vi "Obtain Session.vi"(0 "Listener ID ()":string, 2 "REx Command":refnum<class "REx Command - Root.lvclass">, 11 "error in (no error)":errorcluster) -> (4 "Listener Session Handle":T1, 6 "REx Command Received":refnum<user-event>, 8 "created new?":bool, 15 "error out":errorcluster)   [LabVIEW 2012, in "REx.lvlib" / "Local Listener Session.lvclass"]
doc: "This function initializes the measurement\n\nPass the function a name to obtain an active measurement handle"
uses:
  Local Listener Session.lvclass
  Typedefs/Session Handle.ctl
  REx Command Root/REx Command - Root.lvclass
  Local Listener Session.lvclass/Local Listener Session.ctl
  Utilities/initialize Session Data.vi
  <userlib>/_Session Fwk/Session - Root.lvclass
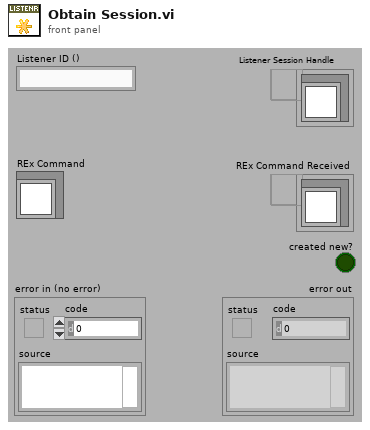
[diagram p1: front panel]
types:
  T1 = typedef "REx.lvlib/Local Listener Session.lvclass/Session Handle.ctl" = refnum<data-value>
  T2 = typedef "Session - Root.lvclass/Session Handle.ctl" = refnum<data-value>
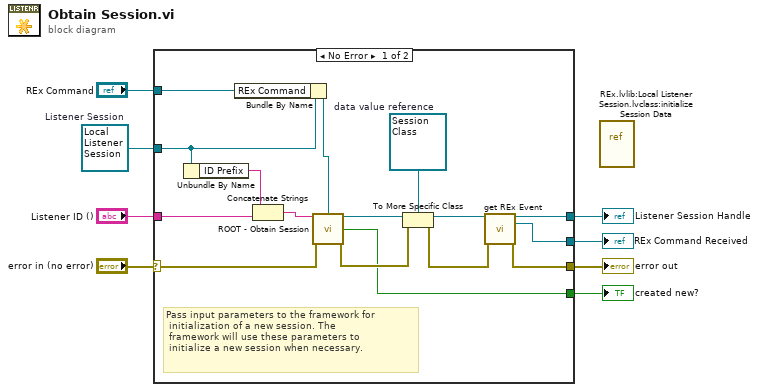
[diagram p0: block diagram]
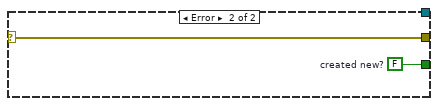
[diagram p2: hidden frame]
diagram:
  w1 = refnum<class "Local Listener Session.lvclass"> refnum  # Listener Session
  n1 = case shown="No Error" "error in (no error)" {
    selector: "error in (no error)" -> [w24 w26]
    tunnel: [w14 w26] -> w7
    tunnel: [w16 _] -> w5
    tunnel: "Listener ID ()" -> [w12 _]
    tunnel: "REx Command" -> [w19 _]
    tunnel: [w18 w25] -> w3
    tunnel: [w13 _] -> w2
    tunnel: w1 -> [w10 _]
    frame No Error {
      w21 = refnum<data-value> refnum  # data value reference
      # "Pass input parameters to the framework for\n initialization of a new session. The\n framework will use these parameters to\n initialize a new session when necessary."
      n2 = Unbundle By Name(w10) -> ("ID Prefix"=w9:string)
      n3 = Bundle By Name(cluster=w10, "REx Command"=w19) -> (w20:refnum<class "Local Listener Session.lvclass">)
      n4 = Concatenate Strings(w9, w12) -> (w11:string)
      n5 = call <userlib>:"ROOT - Obtain Session.vi"("Session Name ()"=w11, "OBJ - Session"=w20, "error in (no error)"=w24) -> ("Session Handle"=w22:T2, "created new?"=w18:bool, "error out"=w23:errorcluster)  [unwired: 10 in]
      n6 = To More Specific Class(target class=w21, reference=w22, error in=w23) -> (specific class reference=w17:refnum<data-value>, error out=w15:errorcluster)
      n7 = call "get REx Event.vi"("Session Handle in"=w17, "error in (no error)"=w15) -> ("Session Handle out"=w16:T1, "Command Event"=w13:refnum<user-event>, "error out"=w14:errorcluster)  [unwired: 11 in]
    }
    frame Error {
      w25 = FALSE  # created new?
    }
  }
  "error out" <- w7
  "Listener Session Handle" <- w5
  "created new?" <- w3
  "REx Command Received" <- w2
  n8 = vi-ref "REx.lvlib:Local Listener Session.lvclass:initialize Session Data.vi"() -> ()  [unwired: 1 out]
